vi "element_to_BSON_bytes.vi"(8 "error in (no error)":errorcluster, 11 "element":variant) -> (0 "error out":errorcluster, 3 "BSONarray":u8[](array[numeric]))   [LabVIEW 2015, in "BSON_convertors_Library.lvlib"]
uses:
  BSON_convertors_Library.lvlib
  <userlib>/_OpenG.lib/lvdata/lvdata.llb/Type Descriptor Enumeration__ogtk.ctl
  typedefs/dataType.ctl
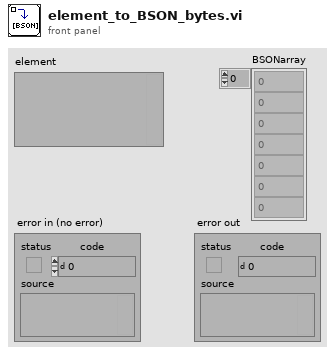
[diagram p1: front panel]
types:
  T1 = typedef "Type Descriptor Enumeration__ogtk.ctl" = enum8{"<Null>", "I8", "I16", "I32", "I64", "U8", "U16", "U32", "U64", "SGL", "DBL", "EXT", "CSG", "CDB", "CXT", "0x0F", "0x10", "0x11", "0x12", "0x13", "0x14", "Enum U8", "Enum U16", "Enum U32", "Enum U64", "SGL PQ", "DBL PQ", "EXT PQ", "CSG PQ", "CDB PQ", "CXT PQ", "0x1F", "0x20", "Boolean", "0x22", "0x23", "0x24", "0x25", "0x26", "0x27", "0x28", "0x29", "0x2A", "0x2B", "0x2C", "0x2D", "0x2E", "0x2F", "String", "0x31", "Path", "Pict", "0x34", "0x35", "0x36", "DAQ", "0x38", "0x39", "0x3A", "0x3B", "0x3C", "0x3D", "0x3E", "0x3F", "Array", "0x41", "0x42", "0x43", "0x44", "0x45", "0x46", "0x47", "0x48", "0x49", "0x4A", "0x4B", "0x4C", "0x4D", "0x4E", "0x4F", "Cluster", "0x51", "0x52", "Variant", "Waveform", "0x55", "0x56", "0x57", "0x58", "0x59", "0x5A", "0x5B", "0x5C", "0x5D", "0x5E", "0x5F", "0x60", "0x61", "0x62", "0x63", "0x64", "0x65", "0x66", "0x67", "0x68", "0x69", "0x6A", "0x6B", "0x6C", "0x6D", "0x6E", "0x6F", "Refnum"}
  T2 = typedef "BSON_convertors_Library.lvlib/dataType.ctl" = enum8{"empty(terminator)", "double", "string", "document", "array", "binary", "Deprecated(Undefined)", "ObjectId", "boolean", "UTC datetime", "Null value", "cstring", "Deprecated(DBPointer)", "JavaScript", "Deprecated(Symbol)", "code_w_s", "int32", "uint64", "int64", "ext (decimal128)", "Min key", "Max key"}
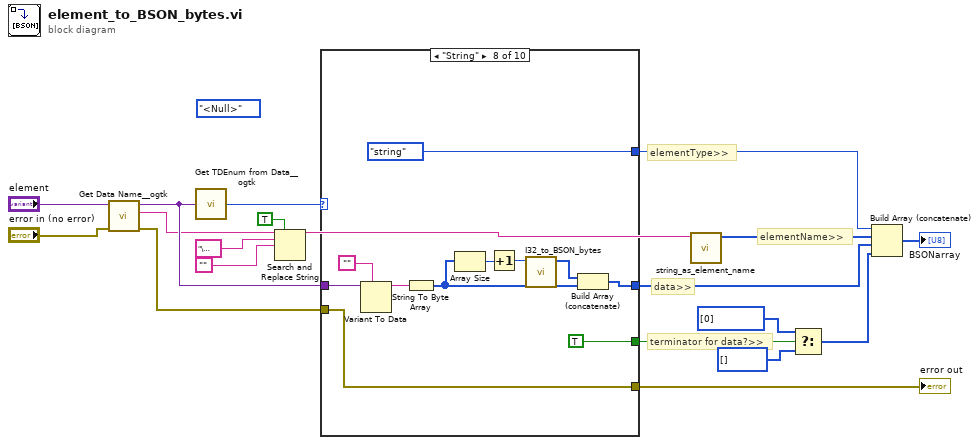
[diagram p0: block diagram]
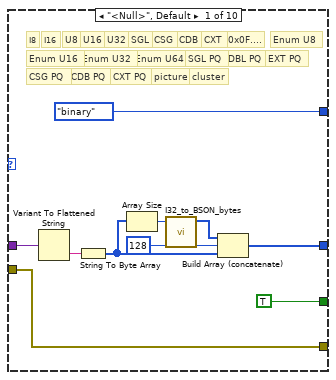
[diagram p2: hidden frame]
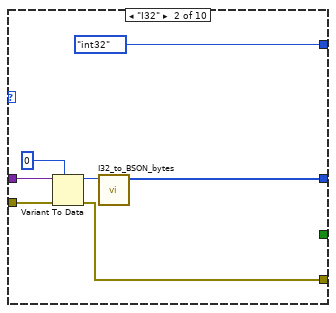
[diagram p3: hidden frame]
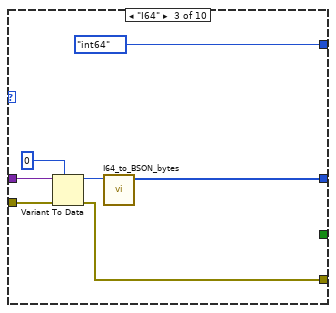
[diagram p4: hidden frame]
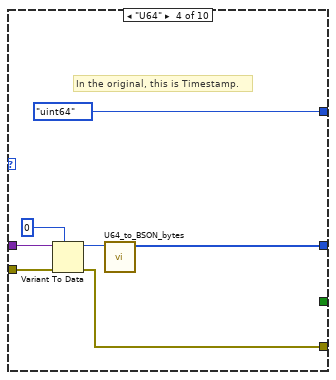
[diagram p5: hidden frame]
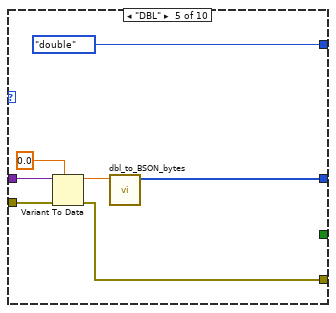
[diagram p6: hidden frame]
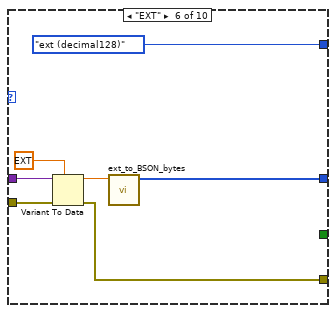
[diagram p7: hidden frame]
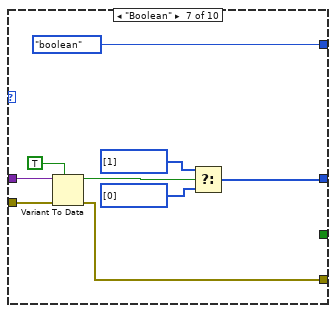
[diagram p8: hidden frame]
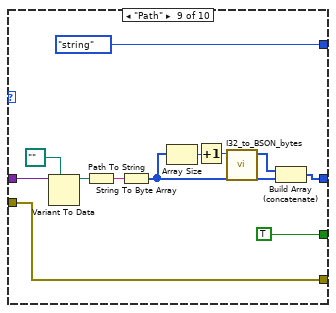
[diagram p9: hidden frame]
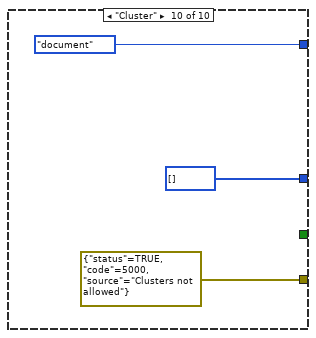
[diagram p10: hidden frame]
diagram:
  (unwired) Type_Descriptor_Enumeration__ogtk."<Null>" ("Type Descriptor Enumeration")
  # "data>>"
  # "elementName>>"
  # "terminator for data?>>"
  # "elementType>>"
  n1 = call <userlib>:"Get Data Name__ogtk.vi"("error in (no error)"="error in (no error)", "Data"="element") -> ("error out"=w10:errorcluster, "Data Name"=w15:string, "Data dup"=w16:variant)  [unwired: 7 in]
  n2 = call <userlib>:"Get TDEnum from Data__ogtk.vi"("Data"=w16) -> ("Type Descriptor Enumeration"=w18:T1)  [unwired: 4 in]
  n3 = Search and Replace String(replace all?=TRUE ("replace all? (F)"), input string=w15, search string="\u0000", replace string="") -> (result string=w14:string)  [unwired: 4 in, 3 out]
  n4 = case shown="\"String\"" w18 {
    tunnel: w16 -> [w29 w35 w42 w49 w56 w63 w72 w77 w89 _]
    tunnel: [dataType."binary" ("dataType") dataType."int32" ("dataType") dataType."int64" ("dataType") dataType."uint64" ("dataType") dataType."double" ("dataType") dataType."ext (decimal128)" ("dataType") dataType."boolean" ("dataType") dataType."string" ("dataType") dataType."string" ("dataType") dataType."document" ("dataType")] -> w6
    tunnel: [TRUE _ _ _ _ _ _ TRUE TRUE _] -> w9
    tunnel: [w21 w30 w37 w44 w51 w58 w65 w79 w91 u8[] [] ("BSONbytes")] -> w4
    tunnel: w10 -> [w20 w32 w40 w47 w54 w61 w71 w78 w90 _]
    tunnel: [w20 w31 w39 w46 w53 w60 w70 w78 w90 errorcluster {"status"=TRUE, "code"=5000, "source"="Clusters not allowed"} ("error out")] -> w1
    frame "<Null>", Default {
      # "cluster"
      # "picture"
      # "CXT PQ"
      # "CDB PQ"
      # "CSG PQ"
      # "EXT PQ"
      # "DBL PQ"
      # "SGL PQ"
      # "Enum U64"
      # "Enum U32"
      # "Enum U16"
      # "Enum U8"
      # "0x0F...."
      # "CXT"
      # "CDB"
      # "CSG"
      # "SGL"
      # "U32"
      # "U16"
      # "U8"
      # "I8"
      # "I16"
      n5 = Variant To Flattened String(Variant=w29) -> (data string=w26:string)  [unwired: 1 out]
      n6 = String To Byte Array(string=w26) -> (unsigned byte array=w22:u8[])
      n7 = Array Size(array=w22) -> (size(s)=w25:i32)
      n8 = call "I32_to_BSON_bytes.vi"("value"=w25) -> ("BSONbytes"=w24:u8[])  [unwired: 10 in]
      n9 = Build Array (concatenate)(w24, u8 128, w22) -> (w21:u8[])
    }
    frame "I32" {
      n10 = Variant To Data(error in=w32, type=0 ("data"), Variant=w35) -> (data=w34:i32, error out=w31:errorcluster)
      n11 = call "I32_to_BSON_bytes.vi"("value"=w34) -> ("BSONbytes"=w30:u8[])  [unwired: 10 in]
    }
    frame "I64" {
      n12 = Variant To Data(error in=w40, type=i64 0 ("data"), Variant=w42) -> (data=w38:i64, error out=w39:errorcluster)
      n13 = call "I64_to_BSON_bytes.vi"("value"=w38) -> ("BSONbytes"=w37:u8[])  [unwired: 10 in]
    }
    frame "U64" {
      # "In the original, this is Timestamp."
      n14 = Variant To Data(error in=w47, type=u64 0 ("data"), Variant=w49) -> (data=w45:u64, error out=w46:errorcluster)
      n15 = call "U64_to_BSON_bytes.vi"("value"=w45) -> ("BSONbytes"=w44:u8[])  [unwired: 10 in]
    }
    frame "DBL" {
      n16 = Variant To Data(error in=w54, type=0.0 ("data"), Variant=w56) -> (data=w52:dbl, error out=w53:errorcluster)
      n17 = call "dbl_to_BSON_bytes.vi"("value"=w52) -> ("BSONbytes"=w51:u8[])  [unwired: 10 in]
    }
    frame "EXT" {
      n18 = Variant To Data(error in=w61, type=ext 0.0 ("data"), Variant=w63) -> (data=w59:ext, error out=w60:errorcluster)
      n19 = call "ext_to_BSON_bytes.vi"("value"=w59) -> ("BSONbytes"=w58:u8[])  [unwired: 10 in]
    }
    frame "Boolean" {
      n20 = Variant To Data(error in=w71, type=TRUE, Variant=w72) -> (data=w68:bool, error out=w70:errorcluster)
      n21 = Select(t=u8[] [1] ("BSONbytes"), s=w68, f=u8[] [0] ("BSONbytes")) -> (s? t:f=w65:u8[])
    }
    frame "String" {
      n22 = Variant To Data(type="", Variant=w77) -> (data=w75:string)  [unwired: 1 in, 1 out]
      n23 = String To Byte Array(string=w75) -> (unsigned byte array=w80:u8[])
      n24 = Array Size(array=w80) -> (size(s)=w82:i32)
      n25 = Increment(x=w82) -> (x+1=w74:i32)
      n26 = call "I32_to_BSON_bytes.vi"("value"=w74) -> ("BSONbytes"=w81:u8[])  [unwired: 10 in]
      n27 = Build Array (concatenate)(w81, w80) -> (w79:u8[])
    }
    frame "Path" {
      n28 = Variant To Data(type=path "", Variant=w89) -> (data=w88:path)  [unwired: 1 in, 1 out]
      n29 = Path To String(path=w88) -> (string=w86:string)
      n30 = String To Byte Array(string=w86) -> (unsigned byte array=w92:u8[])
      n31 = Array Size(array=w92) -> (size(s)=w94:i32)
      n32 = Increment(x=w94) -> (x+1=w85:i32)
      n33 = call "I32_to_BSON_bytes.vi"("value"=w85) -> ("BSONbytes"=w93:u8[])  [unwired: 10 in]
      n34 = Build Array (concatenate)(w93, w92) -> (w91:u8[])
    }
    frame "Cluster" {
    }
  }
  "error out" <- w1
  n35 = call "string_as_element_name.vi"("result string"=w14) -> ("Array"=w5:u8[])  [unwired: 10 in]
  n36 = Select(t=u8[] [0] ("BSONbytes"), s=w9, f=u8[] []) -> (s? t:f=w3:u8[])
  n37 = Build Array (concatenate)(w6, w5, w4, w3) -> (→"BSONarray":u8[])
